vi "Interpolate 2D (1d X,Y).vi"(4 "ntimes":i32=1, 6 "yi":dbl[][](array[numeric]), 7 "method":i32(ring)=1 items=["nearest", "bilinear", "bicubic", "bicubic spline"], 8 "xi":dbl[][](array[numeric]), 9 "Y":dbl[](array[numeric]), 10 "X":dbl[](array[numeric]), 11 "Z":dbl[][](array[numeric])) -> (0 "error":i32, 1 "yi used":dbl[][](array[numeric]), 2 "xi used":dbl[][](array[numeric]), 3 "zi":dbl[][](array[numeric]))   [LabVIEW 2018, in "NI_Gmath.lvlib"]
doc: "Performs two-dimensional interpolation using a selected interpolation method based on the lookup table defined by <B>X</B>, <B>Y</B>, and <B>Z</B>, where <B>Z</B> is a 2D array. You must manually select the polymorphic instance to use."
uses:
  NI_Gmath.lvlib
panel:
  # "Interpolate 2D (1d X,Y)"
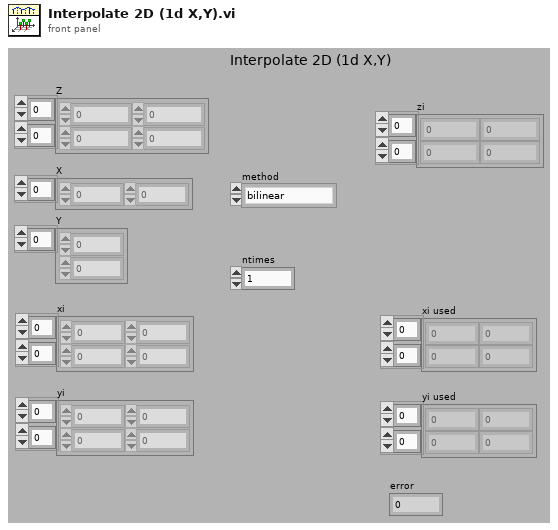
[diagram p1: front panel]
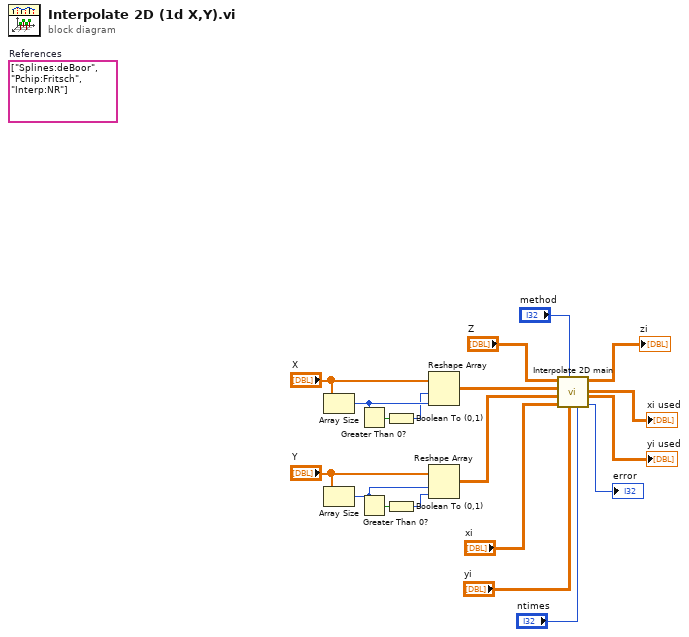
[diagram p0: block diagram]
diagram:
  (unwired) string[] ["Splines:deBoor", "Pchip:Fritsch", "Interp:NR"]  # References
  n1 = Array Size(array="X") -> (size(s)=w10:i32)
  n2 = Array Size(array="Y") -> (size(s)=w6:i32)
  n3 = Greater Than 0?(x=w10) -> (x > 0?=w8:bool)
  n4 = Greater Than 0?(x=w6) -> (x > 0?=w5:bool)
  n5 = Boolean To (0,1)(Boolean=w8) -> (0, 1=w9:i16)
  n6 = Boolean To (0,1)(Boolean=w5) -> (0, 1=w7:i16)
  n7 = Reshape Array("X", w9, w10) -> (w2:dbl[][])
  n8 = Reshape Array("Y", w6, w7) -> (w1:dbl[][])
  n9 = call "Interpolate 2D main.vi"("ntimes"="ntimes", "yi"="yi", "method"="method", "xi"="xi", "Y"=w1, "X"=w2, "Z"="Z") -> ("error"=→"error":i32, "yi used"=→"yi used":dbl[][], "xi used"=→"xi used":dbl[][], "zi"=→"zi":dbl[][])  [unwired: 1 in]
